vi "Write lvlibretls server listener.vi"(8 "error in":errorcluster, 10 "lvlibretls server listener":refnum<class "lvlibretls server listener.lvclass">, 11 "TLS HTTP server in":refnum<class "Basic HTTPS server.lvclass">) -> (0 "error out":errorcluster, 3 "TLS HTTP server out":refnum<class "Basic HTTPS server.lvclass">)   [LabVIEW 2016, in "Basic HTTPS server.lvclass"]
uses:
  Basic HTTPS server.lvclass
  lvlibtls/server/lvlibretls server listener.lvclass
  Basic HTTPS server.lvclass/Basic HTTPS server.ctl
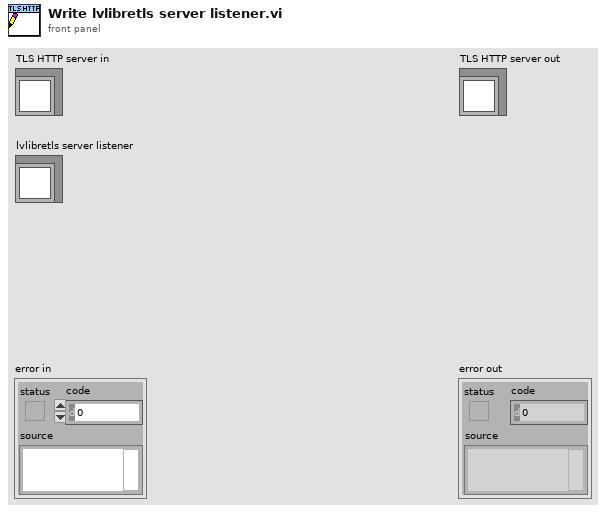
[diagram p1: front panel]
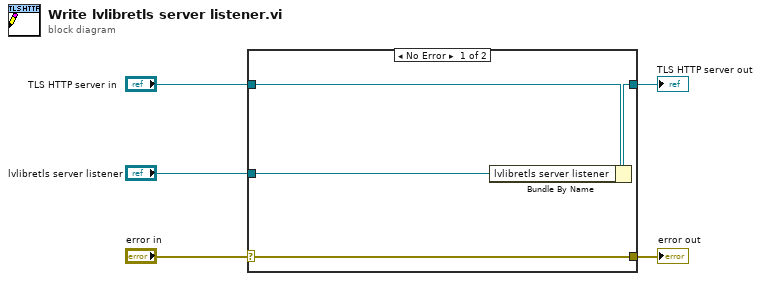
[diagram p0: block diagram]
diagram:
  n1 = case shown="No Error" "error in" {
    selector: "error in" -> [w9 w10]
    tunnel: [w9 w10] -> w4
    tunnel: [w7 w11] -> w2
    tunnel: "TLS HTTP server in" -> [w8 w11]
    tunnel: "lvlibretls server listener" -> [w6 _]
    frame No Error {
      n2 = Bundle By Name(cluster=w8, "lvlibretls server listener"=w6) -> (w7:refnum<class "Basic HTTPS server.lvclass">)
    }
    frame Error {
    }
  }
  "error out" <- w4
  "TLS HTTP server out" <- w2
